vi "Payload to Bit Array.vi"(3 "Payload":string) -> (1 "Bit Array":bool[](array[boolean]))   [LabVIEW 2019]
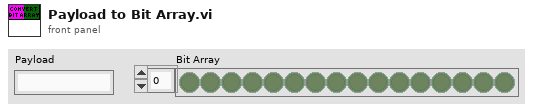
[diagram p1: front panel]
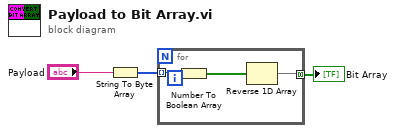
[diagram p0: block diagram]
diagram:
  n1 = String To Byte Array(string="Payload") -> (unsigned byte array=w2:u8[])
  n2 = for {
    tunnel: w2 -> [w6] mode=indexing
    tunnel: [w4] -> w1 mode=concatenating
    n3 = Number To Boolean Array(number=w6) -> (Boolean array=w5:bool[])
    n4 = Reverse 1D Array(array=w5) -> (reversed array=w4:bool[])
  }
  "Bit Array" <- w1
